vi "HMI_FileSaveAs.vi"(11 "File Info":T1) -> (3 "selected path":path)   [LabVIEW 2024]
uses:
  Control Definitions/DEF_ConfigRings.ctl
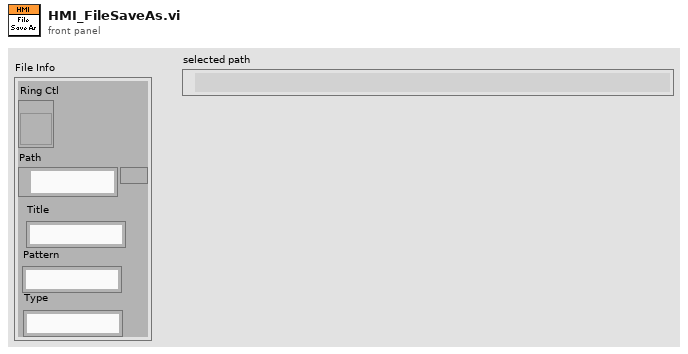
[diagram p1: front panel]
types:
  T1 = typedef "DEF_ConfigRings.ctl" = cluster{"Ring Ctl":refnum<vi>, "Path":path, "Title":string, "Pattern":string, "Type":string}
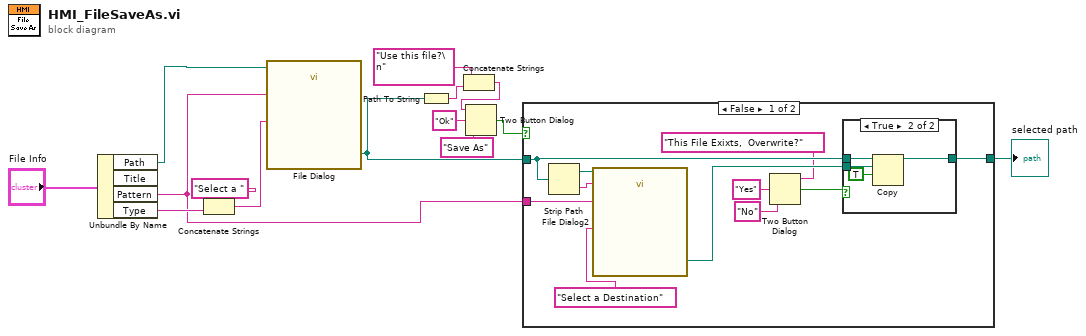
[diagram p0: block diagram]
diagram:
  n1 = Unbundle By Name("File Info") -> ("Path"=w2:path, "Pattern"=w1:string, "Type"=w3:string)  [unwired: 1 out]
  n2 = Concatenate Strings("Select a " ("prompt"), w3) -> (w4:string)
  n3 = call "File Dialog"("start path"=w2, "prompt"=w4, "pattern (all files)"=w1) -> ("selected path"=w11:path)  [unwired: 9 in, 3 out]
  n4 = Path To String(path=w11) -> (string=w9:string)
  n5 = Concatenate Strings("Use this file?\n" ("message"), w9) -> (w8:string)
  n6 = Two Button Dialog(message=w8, 1:"Save As" ("F button name (\"Cancel\")"), 2:"Ok" ("T button name (\"OK\")")) -> (T button?=w7:bool)
  n7 = case shown="False" w7 {
    tunnel: [w25 w31] -> w14
    tunnel: w11 -> [w20 w31]
    tunnel: w1 -> [w15 _]
    frame False {
      n8 = Strip Path(path=w20) -> (stripped path=w24:path, name=w23:string)
      n9 = call "File Dialog2"("start path"=w24, "prompt"="Select a Destination", "default name"=w23, "pattern (all files)"=w15) -> ("selected path"=w22:path)  [unwired: 8 in, 3 out]
      n10 = Two Button Dialog(message="This File Exixts,  Overwrite?", 1:"No" ("F button name (\"Cancel\")"), 2:"Yes" ("T button name (\"OK\")")) -> (T button?=w16:bool)
      n11 = case shown="True" w16 {
        tunnel: [w26 w30] -> w25
        tunnel: w22 -> [_ w29]
        tunnel: w20 -> [w26 w28]
        frame False {
        }
        frame True {
          n12 = Copy(9:TRUE ("overwrite (F)"), 10:w29, 11:w28) -> (3:w30:path)  [unwired: 2 in, 2 out]
        }
      }
    }
    frame True {
    }
  }
  "selected path" <- w14
